vi "tp7 remp.vi"() -> ()   [LabVIEW 2017]
uses:
  enum_Etats.ctl
panel:
  out "Bouteille bouchée":u8(slide) scale=0.0..100.0
  out "Nombre de bouteilles":dbl format="%#g"
  in  "bouteille vide":u8(slide) scale=0.0..100.0
  out "Bouteille Remlpie":dbl
  out "vérin v2":u8(slide) scale=0.0..100.0
  out "vérin v1":u8(slide) scale=0.0..100.0
  out "Poste de bouchage":u8(slide)
  out "Poste de remlissage":u8(slide) scale=0.0..100.0
  out "d22":bool
  in  "d21":bool
  out "d12":bool
  out "d11":bool
  in  "arret d'urgence":bool
  in  "marche/arret":bool
  # "Interface de supervision et de commande d'une ligne d'embouteillage"
  # "Buse"
  # "Verin V3"
  # "Arrivée des Bouteilles"
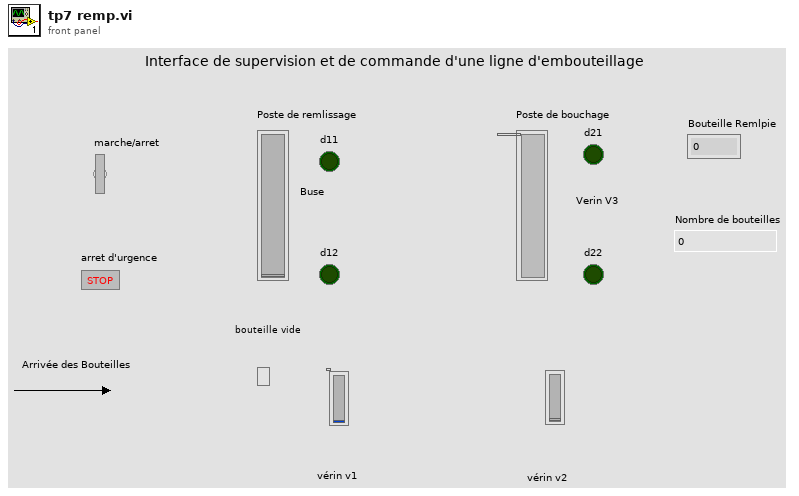
[diagram p1: front panel]
types:
  T1 = typedef "enum_Etats.ctl" = enum16{"Intialisation", "Dép Remplisaage", "Dep Bouchage", "Remlpissage", "Bouchage"}
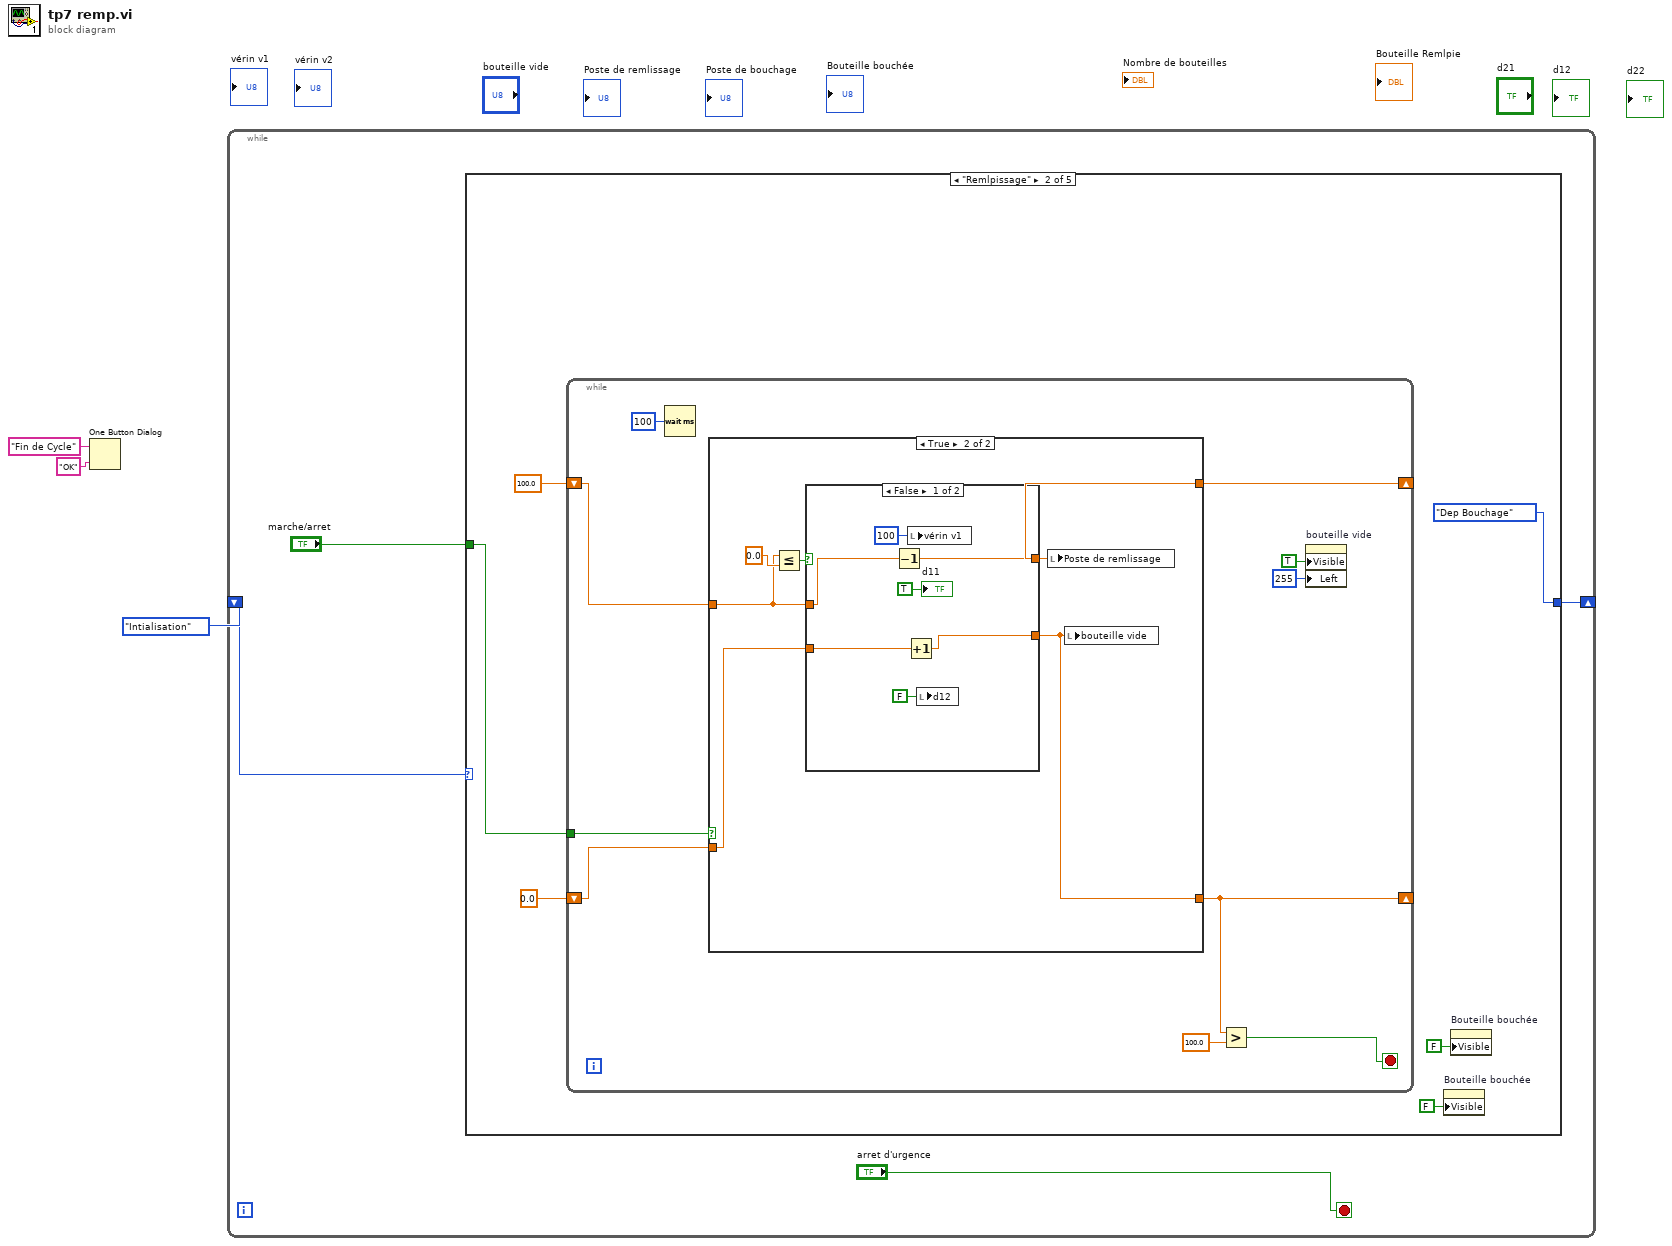
[diagram p0: block diagram]
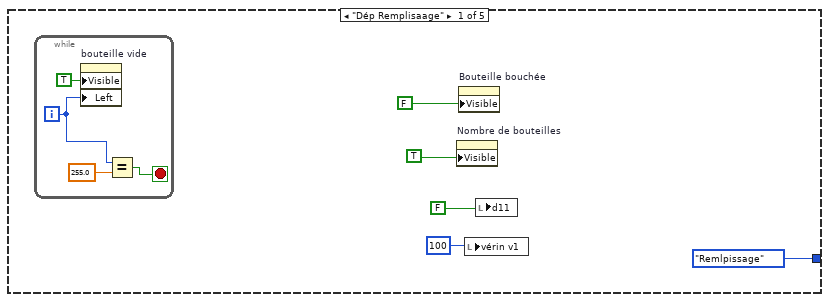
[diagram p2: hidden frame]
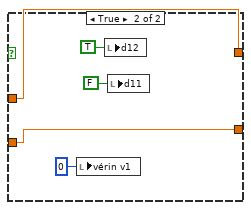
[diagram p4: hidden frame]
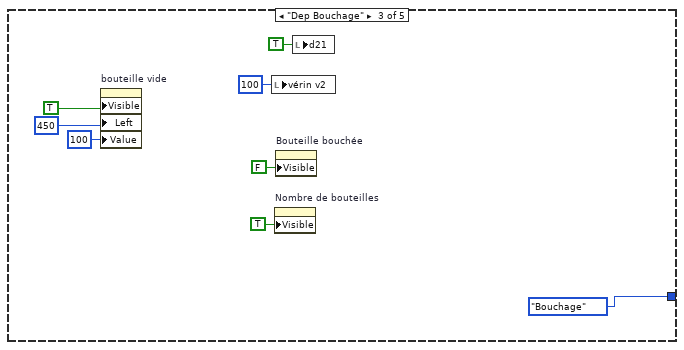
[diagram p5: hidden frame]
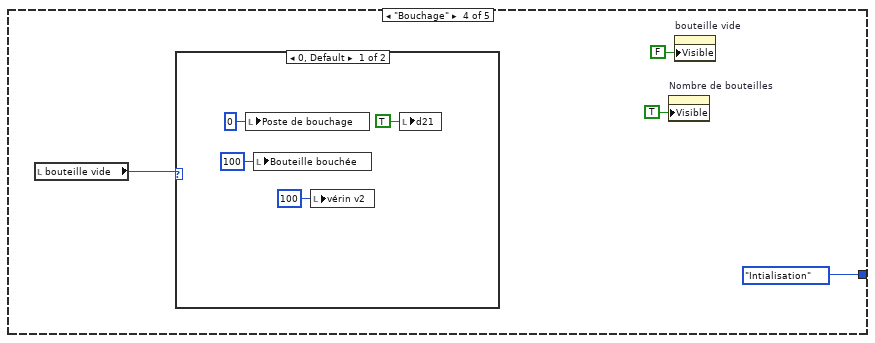
[diagram p6: hidden frame]
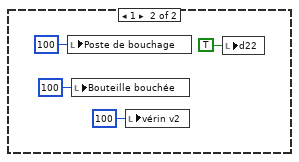
[diagram p7: hidden frame]
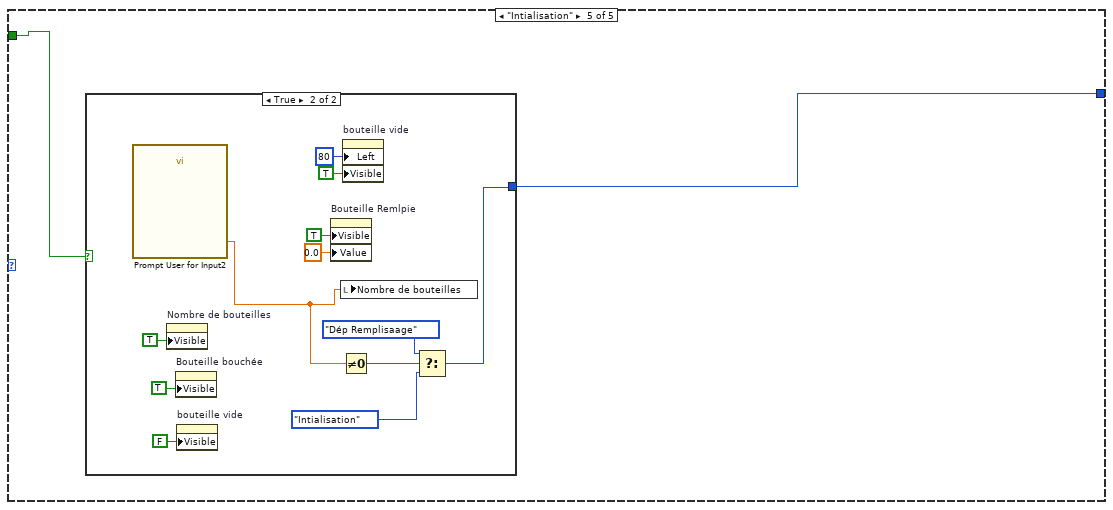
[diagram p8: hidden frame]
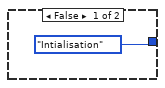
[diagram p9: hidden frame]
diagram:
  n1 = One Button Dialog(message="Fin de Cycle", button name ("OK")="OK") -> ()  [unwired: 1 out]
  n2 = while {
    shift-right: [w6] -> _
    shift-left: enum_Etats."Intialisation" -> [w5]
    stop <- "arret d'urgence" stop-if-true
    n3 = case shown="\"Remlpissage\"" w5 {
      tunnel: "marche/arret" -> [_ w19 _ _ w73]
      tunnel: [enum_Etats."Remlpissage" enum_Etats."Dep Bouchage" enum_Etats."Bouchage" enum_Etats."Intialisation" w74] -> w6
      frame "Dép Remplisaage" {
        n4 = while {
          i -> [w13]
          stop <- w15 stop-if-true
          n5 = property on="bouteille vide" class="Slide (strict)"("Visible"=TRUE, "Left"=w13) -> ()  [unwired: 2 in, 2 out]
          n6 = Equal?(x=w13, y=255.0) -> (x = y?=w15:bool)
        }
        n7 = property on="Nombre de bouteilles" class="DigNum (strict)"("Visible"=TRUE) -> ()  [unwired: 2 in, 2 out]
        n8 = property on="Bouteille bouchée" class="Slide (strict)"("Visible"=FALSE) -> ()  [unwired: 2 in, 2 out]
        n9 = local write "vérin v1"(u8 100 ("vérin v1")) -> ()
        n10 = local write "d11"(FALSE ("d11")) -> ()
      }
      frame "Remlpissage" {
        n11 = while {
          shift-right: [w28] -> _
          shift-left: 100.0 ("x") -> [w30]
          tunnel: w19 -> [w26]
          shift-right: [w24] -> _
          shift-left: 0.0 ("y") -> [w29]
          stop <- w25 stop-if-true
          n12 = Wait (ms)(milliseconds to wait=u32 100) -> ()  [unwired: 1 out]
          n13 = case shown="True" w26 {
            tunnel: w30 -> [w34 w37]
            tunnel: w29 -> [w33 w36]
            tunnel: [w34 w39] -> w28
            tunnel: [w33 w35] -> w24
            frame False {
            }
            frame True {
              n14 = Less Or Equal?(x=w37, y=0.0 ("x")) -> (x <= y?=w40:bool)
              n15 = case shown="False" w40 {
                tunnel: [w45 w52] -> w39
                tunnel: w37 -> [w44 w52]
                tunnel: w36 -> [w43 w49]
                tunnel: [w41 w49] -> w35
                frame False {
                  n16 = Decrement(x=w44) -> (x-1=w45:dbl)
                  n17 = Increment(x=w43) -> (x+1=w41:dbl)
                  n18 = local write "vérin v1"(u8 100 ("vérin v1")) -> ()
                  n19 = local write "d12"(FALSE ("d12")) -> ()
                  "d11" <- TRUE ("d11")
                }
                frame True {
                  n20 = local write "vérin v1"(u8 0 ("vérin v1")) -> ()
                  n21 = local write "d12"(TRUE ("d12")) -> ()
                  n22 = local write "d11"(FALSE ("d12")) -> ()
                }
              }
              n23 = local write "Poste de remlissage"(w39) -> ()
              n24 = local write "bouteille vide"(w35) -> ()
            }
          }
          n25 = Greater?(x=w24, y=100.0) -> (0:w25:bool)
          n26 = property on="bouteille vide" class="Slide (strict)"("Visible"=TRUE, "Left"=255 ("Position:Left")) -> ()  [unwired: 2 in, 2 out]
        }
        n27 = property on="Bouteille bouchée" class="Slide (strict)"("Visible"=FALSE) -> ()  [unwired: 2 in, 2 out]
        n28 = property on="Bouteille bouchée" class="Slide (strict)"("Visible"=FALSE) -> ()  [unwired: 2 in, 2 out]
      }
      frame "Dep Bouchage" {
        n29 = property on="bouteille vide" class="Slide (strict)"("Visible"=TRUE, "Left"=450 ("Position:Left"), "Value"=u8 100 ("bouteille vide")) -> ()  [unwired: 2 in, 2 out]
        n30 = local write "vérin v2"(u8 100 ("vérin v2")) -> ()
        n31 = property on="Nombre de bouteilles" class="DigNum (strict)"("Visible"=TRUE) -> ()  [unwired: 2 in, 2 out]
        n32 = property on="Bouteille bouchée" class="Slide (strict)"("Visible"=FALSE) -> ()  [unwired: 2 in, 2 out]
        n33 = local write "d21"(TRUE ("d21")) -> ()
      }
      frame "Bouchage" {
        n34 = local read "bouteille vide"() -> (w63:u8)
        n35 = case shown="0, Default" w63 {
          frame 0, Default {
            n36 = local write "Poste de bouchage"(u8 0 ("Poste de bouchage")) -> ()
            n37 = local write "Bouteille bouchée"(u8 100 ("Bouteille bouchée")) -> ()
            n38 = local write "vérin v2"(u8 100 ("vérin v2")) -> ()
            n39 = local write "d21"(TRUE ("d12")) -> ()
          }
          frame 1 {
            n40 = local write "Poste de bouchage"(u8 100 ("Poste de bouchage")) -> ()
            n41 = local write "Bouteille bouchée"(u8 100 ("Bouteille bouchée")) -> ()
            n42 = local write "vérin v2"(u8 100 ("vérin v2")) -> ()
            n43 = local write "d22"(TRUE ("d22")) -> ()
          }
        }
        n44 = property on="Nombre de bouteilles" class="DigNum (strict)"("Visible"=TRUE) -> ()  [unwired: 2 in, 2 out]
        n45 = property on="bouteille vide" class="Slide (strict)"("Visible"=FALSE) -> ()  [unwired: 2 in, 2 out]
      }
      frame "Intialisation" {
        n46 = case shown="True" w73 {
          tunnel: [enum_Etats."Intialisation" w80] -> w74
          frame False {
          }
          frame True {
            n47 = call "Prompt User for Input2"() -> ("nombere de bouteilles"=w77:dbl)  [unwired: 17 in, 2 out]
            n48 = property on="Nombre de bouteilles" class="DigNum (strict)"("Visible"=TRUE) -> ()  [unwired: 2 in, 2 out]
            n49 = property on="Bouteille bouchée" class="Slide (strict)"("Visible"=TRUE) -> ()  [unwired: 2 in, 2 out]
            n50 = property on="bouteille vide" class="Slide (strict)"("Visible"=FALSE) -> ()  [unwired: 2 in, 2 out]
            n51 = property on="Bouteille Remlpie" class="DigNum (strict)"("Visible"=TRUE, "Value"=0.0 ("Bouteille Remlpie")) -> ()  [unwired: 2 in, 2 out]
            n52 = local write "Nombre de bouteilles"(w77) -> ()
            n53 = Not Equal To 0?(x=w77) -> (x != 0?=w83:bool)
            n54 = property on="bouteille vide" class="Slide (strict)"("Left"=80 ("Position:Left"), "Visible"=TRUE) -> ()  [unwired: 2 in, 2 out]
            n55 = Select(t=enum_Etats."Dép Remplisaage", s=w83, f=enum_Etats."Intialisation") -> (s? t:f=w80:T1)
          }
        }
      }
    }
  }
